vi "Elimina acquisizione.vi"(8 "indice prova":i32, 9 "indice riga":i32, 10 "tabella":i32, 11 "Dati prove in 2":T1) -> (1 "riga eliminata":string[](array[string]), 3 "Dati prove out 3":T1)   [LabVIEW 2019]
uses:
  TypeDef/Dati collaudo.ctl
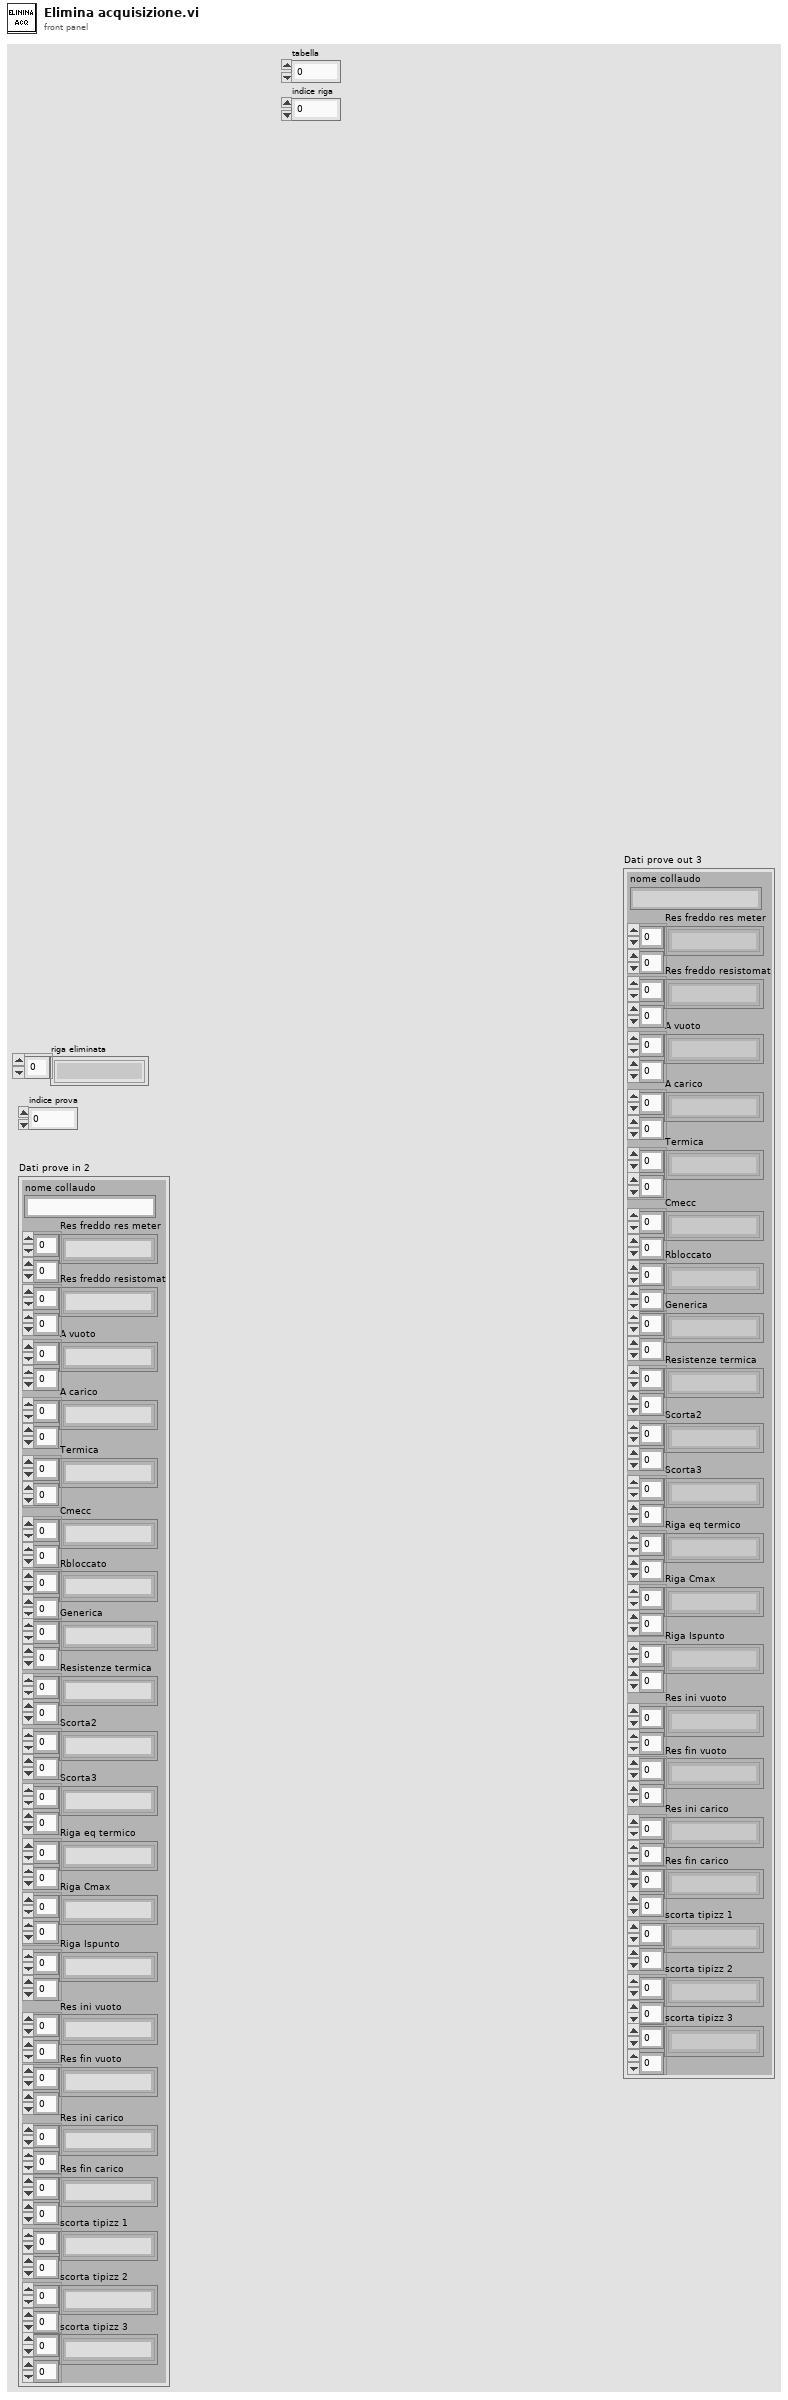
[diagram p1: front panel]
types:
  T1 = typedef "Dati collaudo.ctl" = cluster{"nome collaudo":string, "Res freddo res meter":string[][], "Res freddo resistomat":string[][], "A vuoto":string[][], "A carico":string[][], "Termica":string[][], "Cmecc":string[][], "Rbloccato":string[][], "Generica":string[][], "Resistenze termica":string[][], "Scorta2":string[][], "Scorta3":string[][], "Riga eq termico":string[][], "Riga Cmax":string[][], "Riga Ispunto":string[][], "Res ini vuoto":string[][], "Res fin vuoto":string[][], "Res ini carico":string[][], "Res fin carico":string[][], "scorta tipizz 1":string[][], "scorta tipizz 2":string[][], "scorta tipizz 3":string[][]}
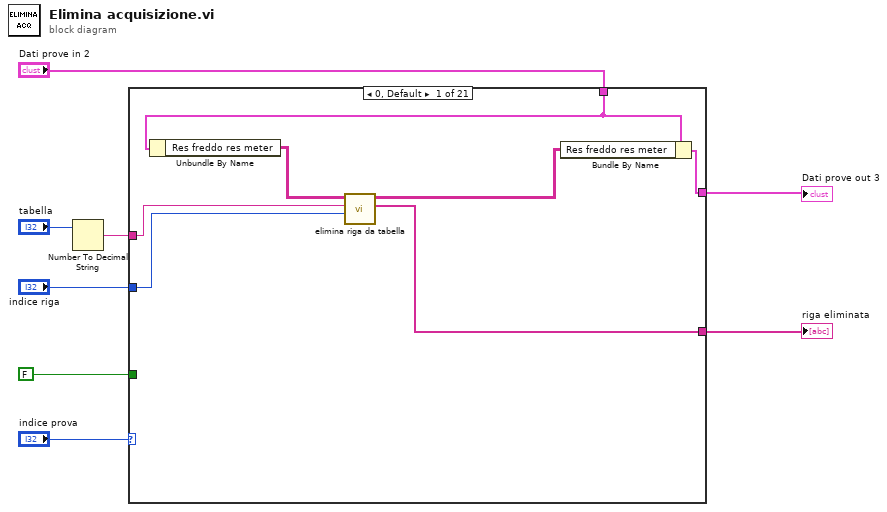
[diagram p0: block diagram]
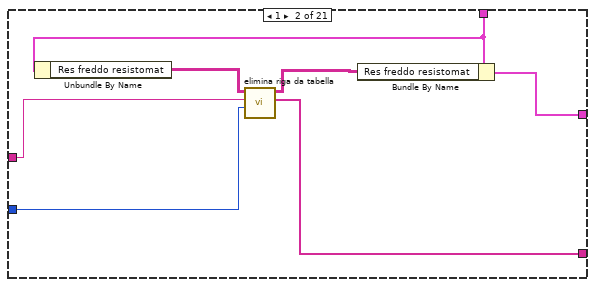
[diagram p2: hidden frame]
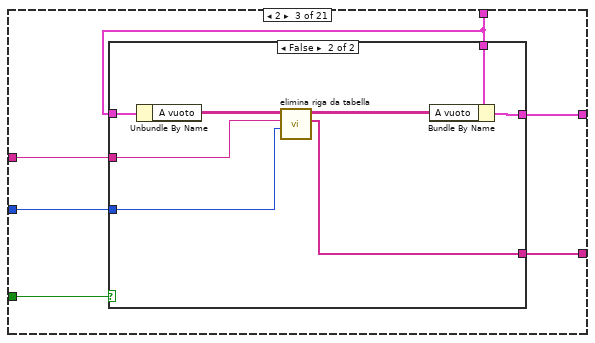
[diagram p3: hidden frame]
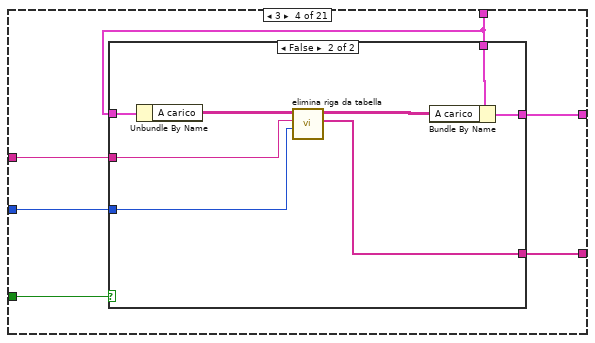
[diagram p5: hidden frame]
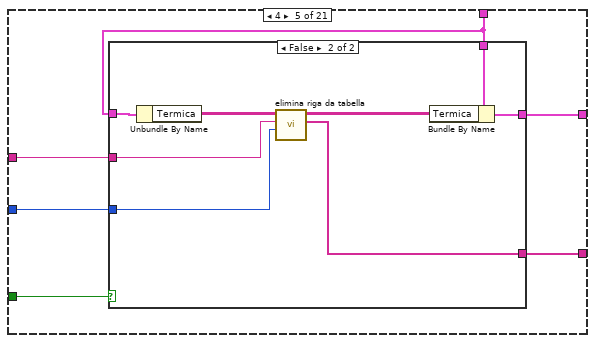
[diagram p7: hidden frame]
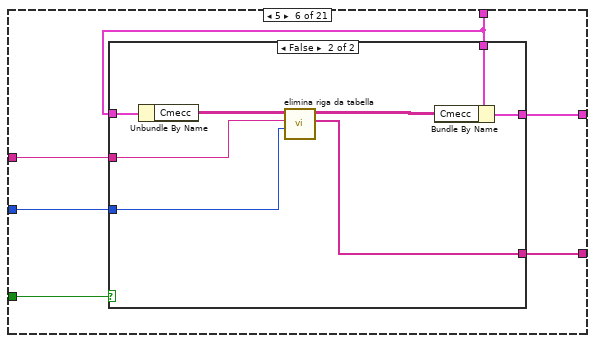
[diagram p9: hidden frame]
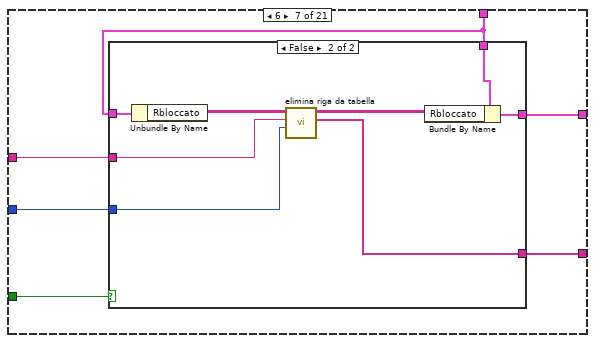
[diagram p11: hidden frame]
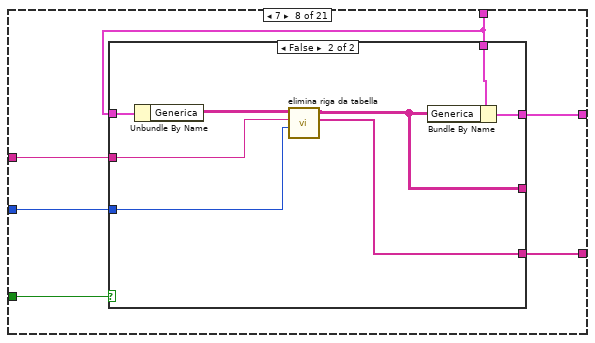
[diagram p13: hidden frame]
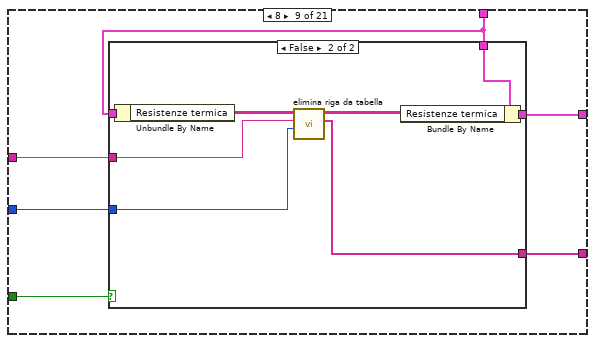
[diagram p15: hidden frame]
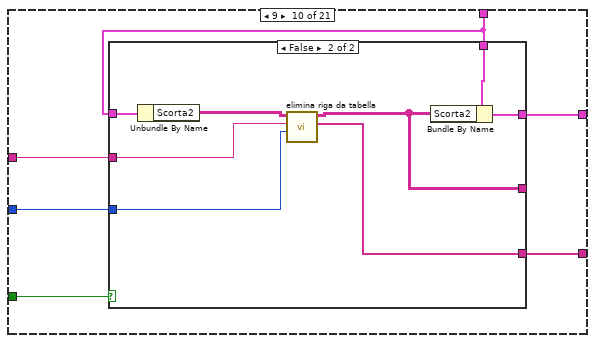
[diagram p17: hidden frame]
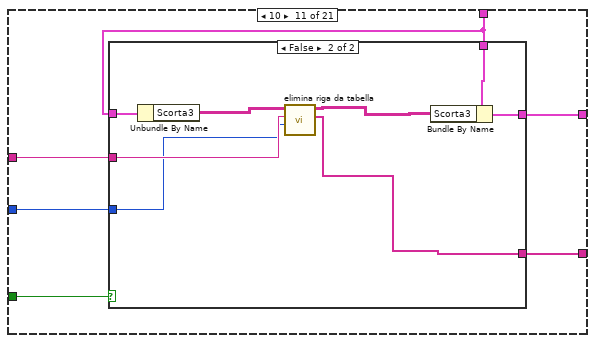
[diagram p19: hidden frame]
diagram:
  n1 = Number To Decimal String(number="tabella") -> (decimal integer string=w3:string)  [unwired: 1 in]
  n2 = case shown="0, Default" "indice prova" {
    tunnel: FALSE -> [_ _ w28 w43 w58 w73 w88 w103 w118 w133 w148 _ _ _ _ _ _ _ _ _ _]
    tunnel: [w15 w22 w27 w42 w57 w72 w87 w102 w117 w132 w147 w164 w171 w178 w185 w192 w199 w206 w213 w220 w227] -> w5
    tunnel: "Dati prove in 2" -> [w14 w21 w26 w41 w56 w71 w86 w101 w116 w131 w146 w163 w170 w177 w184 w191 w198 w205 w212 w219 w226]
    tunnel: [w9 w18 w25 w40 w55 w70 w85 w100 w115 w130 w145 w159 w167 w174 w180 w188 w193 w202 w207 w214 w221] -> w8
    tunnel: w3 -> [w12 w17 w24 w39 w54 w69 w84 w99 w114 w129 w144 w160 w166 w173 w181 w187 w195 w201 w209 w216 w223]
    tunnel: "indice riga" -> [w11 w16 w23 w38 w53 w68 w83 w98 w113 w128 w143 w158 w165 w172 w179 w186 w194 w200 w208 w215 w222]
    frame 0, Default {
      n3 = Unbundle By Name(w14) -> ("Res freddo res meter"=w13:string[][])
      n4 = call "elimina riga da tabella.vi"("indice riga"=w11, "tab"=w12, "Res freddo res meter in"=w13) -> ("riga eliminata"=w9:string[], "Array"=w10:string[][])  [unwired: 7 in]
      n5 = Bundle By Name(cluster=w14, "Res freddo res meter"=w10) -> (w15:T1)
    }
    frame 1 {
      n6 = Unbundle By Name(w21) -> ("Res freddo resistomat"=w20:string[][])
      n7 = call "elimina riga da tabella.vi"("indice riga"=w16, "tab"=w17, "Res freddo res meter in"=w20) -> ("riga eliminata"=w18:string[], "Array"=w19:string[][])  [unwired: 7 in]
      n8 = Bundle By Name(cluster=w21, "Res freddo resistomat"=w19) -> (w22:T1)
    }
    frame 2 {
      n9 = case shown="False" w28 {
        tunnel: [w29 w37] -> w27
        tunnel: w26 -> [w29 w36]
        tunnel: w26 -> [_ w35]
        tunnel: [_ w30] -> w25
        tunnel: w24 -> [_ w32]
        tunnel: w23 -> [_ w31]
        frame True {
        }
        frame False {
          n10 = Unbundle By Name(w35) -> ("A vuoto"=w34:string[][])
          n11 = call "elimina riga da tabella.vi"("indice riga"=w31, "tab"=w32, "Res freddo res meter in"=w34) -> ("riga eliminata"=w30:string[], "Array"=w33:string[][])  [unwired: 7 in]
          n12 = Bundle By Name(cluster=w36, "A vuoto"=w33) -> (w37:T1)
        }
      }
    }
    frame 3 {
      n13 = case shown="False" w43 {
        tunnel: [w44 w52] -> w42
        tunnel: w41 -> [w44 w51]
        tunnel: w41 -> [_ w50]
        tunnel: [_ w45] -> w40
        tunnel: w39 -> [_ w47]
        tunnel: w38 -> [_ w46]
        frame True {
        }
        frame False {
          n14 = Unbundle By Name(w50) -> ("A carico"=w49:string[][])
          n15 = call "elimina riga da tabella.vi"("indice riga"=w46, "tab"=w47, "Res freddo res meter in"=w49) -> ("riga eliminata"=w45:string[], "Array"=w48:string[][])  [unwired: 7 in]
          n16 = Bundle By Name(cluster=w51, "A carico"=w48) -> (w52:T1)
        }
      }
    }
    frame 4 {
      n17 = case shown="False" w58 {
        tunnel: [w59 w67] -> w57
        tunnel: w56 -> [w59 w66]
        tunnel: w56 -> [_ w65]
        tunnel: [_ w60] -> w55
        tunnel: w54 -> [_ w62]
        tunnel: w53 -> [_ w61]
        frame True {
        }
        frame False {
          n18 = Unbundle By Name(w65) -> ("Termica"=w64:string[][])
          n19 = call "elimina riga da tabella.vi"("indice riga"=w61, "tab"=w62, "Res freddo res meter in"=w64) -> ("riga eliminata"=w60:string[], "Array"=w63:string[][])  [unwired: 7 in]
          n20 = Bundle By Name(cluster=w66, "Termica"=w63) -> (w67:T1)
        }
      }
    }
    frame 5 {
      n21 = case shown="False" w73 {
        tunnel: [w74 w82] -> w72
        tunnel: w71 -> [w74 w81]
        tunnel: w71 -> [_ w80]
        tunnel: [_ w75] -> w70
        tunnel: w69 -> [_ w77]
        tunnel: w68 -> [_ w76]
        frame True {
        }
        frame False {
          n22 = Unbundle By Name(w80) -> ("Cmecc"=w79:string[][])
          n23 = call "elimina riga da tabella.vi"("indice riga"=w76, "tab"=w77, "Res freddo res meter in"=w79) -> ("riga eliminata"=w75:string[], "Array"=w78:string[][])  [unwired: 7 in]
          n24 = Bundle By Name(cluster=w81, "Cmecc"=w78) -> (w82:T1)
        }
      }
    }
    frame 6 {
      n25 = case shown="False" w88 {
        tunnel: [w89 w97] -> w87
        tunnel: w86 -> [w89 w96]
        tunnel: w86 -> [_ w95]
        tunnel: [_ w90] -> w85
        tunnel: w84 -> [_ w92]
        tunnel: w83 -> [_ w91]
        frame True {
        }
        frame False {
          n26 = Unbundle By Name(w95) -> ("Rbloccato"=w94:string[][])
          n27 = call "elimina riga da tabella.vi"("indice riga"=w91, "tab"=w92, "Res freddo res meter in"=w94) -> ("riga eliminata"=w90:string[], "Array"=w93:string[][])  [unwired: 7 in]
          n28 = Bundle By Name(cluster=w96, "Rbloccato"=w93) -> (w97:T1)
        }
      }
    }
    frame 7 {
      n29 = case shown="False" w103 {
        tunnel: [_ w108] -> _
        tunnel: [w104 w112] -> w102
        tunnel: w101 -> [w104 w111]
        tunnel: w101 -> [_ w110]
        tunnel: [_ w106] -> w100
        tunnel: w99 -> [_ w107]
        tunnel: w98 -> [_ w105]
        frame True {
        }
        frame False {
          n30 = Unbundle By Name(w110) -> ("Generica"=w109:string[][])
          n31 = call "elimina riga da tabella.vi"("indice riga"=w105, "tab"=w107, "Res freddo res meter in"=w109) -> ("riga eliminata"=w106:string[], "Array"=w108:string[][])  [unwired: 7 in]
          n32 = Bundle By Name(cluster=w111, "Generica"=w108) -> (w112:T1)
        }
      }
    }
    frame 8 {
      n33 = case shown="False" w118 {
        tunnel: [w119 w127] -> w117
        tunnel: w116 -> [w119 w126]
        tunnel: w116 -> [_ w125]
        tunnel: [_ w121] -> w115
        tunnel: w114 -> [_ w122]
        tunnel: w113 -> [_ w120]
        frame True {
        }
        frame False {
          n34 = Unbundle By Name(w125) -> ("Resistenze termica"=w124:string[][])
          n35 = call "elimina riga da tabella.vi"("indice riga"=w120, "tab"=w122, "Res freddo res meter in"=w124) -> ("riga eliminata"=w121:string[], "Array"=w123:string[][])  [unwired: 7 in]
          n36 = Bundle By Name(cluster=w126, "Resistenze termica"=w123) -> (w127:T1)
        }
      }
    }
    frame 9 {
      n37 = case shown="False" w133 {
        tunnel: [_ w138] -> _
        tunnel: [w134 w142] -> w132
        tunnel: w131 -> [w134 w141]
        tunnel: w131 -> [_ w140]
        tunnel: [_ w136] -> w130
        tunnel: w129 -> [_ w137]
        tunnel: w128 -> [_ w135]
        frame True {
        }
        frame False {
          n38 = Unbundle By Name(w140) -> ("Scorta2"=w139:string[][])
          n39 = call "elimina riga da tabella.vi"("indice riga"=w135, "tab"=w137, "Res freddo res meter in"=w139) -> ("riga eliminata"=w136:string[], "Array"=w138:string[][])  [unwired: 7 in]
          n40 = Bundle By Name(cluster=w141, "Scorta2"=w138) -> (w142:T1)
        }
      }
    }
    frame 10 {
      n41 = case shown="False" w148 {
        tunnel: [w149 w157] -> w147
        tunnel: w146 -> [w149 w156]
        tunnel: w146 -> [_ w155]
        tunnel: [_ w151] -> w145
        tunnel: w144 -> [_ w152]
        tunnel: w143 -> [_ w150]
        frame True {
        }
        frame False {
          n42 = Unbundle By Name(w155) -> ("Scorta3"=w154:string[][])
          n43 = call "elimina riga da tabella.vi"("indice riga"=w150, "tab"=w152, "Res freddo res meter in"=w154) -> ("riga eliminata"=w151:string[], "Array"=w153:string[][])  [unwired: 7 in]
          n44 = Bundle By Name(cluster=w156, "Scorta3"=w153) -> (w157:T1)
        }
      }
    }
    frame 11 {
      n45 = Unbundle By Name(w163) -> ("Riga eq termico"=w162:string[][])
      n46 = call "elimina riga da tabella.vi"("indice riga"=w158, "tab"=w160, "Res freddo res meter in"=w162) -> ("riga eliminata"=w159:string[], "Array"=w161:string[][])  [unwired: 7 in]
      n47 = Bundle By Name(cluster=w163, "Riga eq termico"=w161) -> (w164:T1)
    }
    frame 12 {
      n48 = Unbundle By Name(w170) -> ("Riga Cmax"=w169:string[][])
      n49 = call "elimina riga da tabella.vi"("indice riga"=w165, "tab"=w166, "Res freddo res meter in"=w169) -> ("riga eliminata"=w167:string[], "Array"=w168:string[][])  [unwired: 7 in]
      n50 = Bundle By Name(cluster=w170, "Riga Cmax"=w168) -> (w171:T1)
    }
    frame 13 {
      n51 = Unbundle By Name(w177) -> ("Riga Ispunto"=w176:string[][])
      n52 = call "elimina riga da tabella.vi"("indice riga"=w172, "tab"=w173, "Res freddo res meter in"=w176) -> ("riga eliminata"=w174:string[], "Array"=w175:string[][])  [unwired: 7 in]
      n53 = Bundle By Name(cluster=w177, "Riga Ispunto"=w175) -> (w178:T1)
    }
    frame 14 {
      n54 = Unbundle By Name(w184) -> ("Res ini vuoto"=w183:string[][])
      n55 = call "elimina riga da tabella.vi"("indice riga"=w179, "tab"=w181, "Res freddo res meter in"=w183) -> ("riga eliminata"=w180:string[], "Array"=w182:string[][])  [unwired: 7 in]
      n56 = Bundle By Name(cluster=w184, "Res ini vuoto"=w182) -> (w185:T1)
    }
    frame 15 {
      n57 = Unbundle By Name(w191) -> ("Res fin vuoto"=w190:string[][])
      n58 = call "elimina riga da tabella.vi"("indice riga"=w186, "tab"=w187, "Res freddo res meter in"=w190) -> ("riga eliminata"=w188:string[], "Array"=w189:string[][])  [unwired: 7 in]
      n59 = Bundle By Name(cluster=w191, "Res fin vuoto"=w189) -> (w192:T1)
    }
    frame 16 {
      n60 = Unbundle By Name(w198) -> ("Res ini carico"=w197:string[][])
      n61 = call "elimina riga da tabella.vi"("indice riga"=w194, "tab"=w195, "Res freddo res meter in"=w197) -> ("riga eliminata"=w193:string[], "Array"=w196:string[][])  [unwired: 7 in]
      n62 = Bundle By Name(cluster=w198, "Res ini carico"=w196) -> (w199:T1)
    }
    frame 17 {
      n63 = Unbundle By Name(w205) -> ("Res fin carico"=w204:string[][])
      n64 = call "elimina riga da tabella.vi"("indice riga"=w200, "tab"=w201, "Res freddo res meter in"=w204) -> ("riga eliminata"=w202:string[], "Array"=w203:string[][])  [unwired: 7 in]
      n65 = Bundle By Name(cluster=w205, "Res fin carico"=w203) -> (w206:T1)
    }
    frame 18 {
      n66 = Unbundle By Name(w212) -> ("scorta tipizz 1"=w211:string[][])
      n67 = call "elimina riga da tabella.vi"("indice riga"=w208, "tab"=w209, "Res freddo res meter in"=w211) -> ("riga eliminata"=w207:string[], "Array"=w210:string[][])  [unwired: 7 in]
      n68 = Bundle By Name(cluster=w212, "scorta tipizz 1"=w210) -> (w213:T1)
    }
    frame 19 {
      n69 = Unbundle By Name(w219) -> ("scorta tipizz 2"=w218:string[][])
      n70 = call "elimina riga da tabella.vi"("indice riga"=w215, "tab"=w216, "Res freddo res meter in"=w218) -> ("riga eliminata"=w214:string[], "Array"=w217:string[][])  [unwired: 7 in]
      n71 = Bundle By Name(cluster=w219, "scorta tipizz 2"=w217) -> (w220:T1)
    }
    frame 20 {
      n72 = Unbundle By Name(w226) -> ("scorta tipizz 3"=w225:string[][])
      n73 = call "elimina riga da tabella.vi"("indice riga"=w222, "tab"=w223, "Res freddo res meter in"=w225) -> ("riga eliminata"=w221:string[], "Array"=w224:string[][])  [unwired: 7 in]
      n74 = Bundle By Name(cluster=w226, "scorta tipizz 3"=w224) -> (w227:T1)
    }
  }
  "Dati prove out 3" <- w5
  "riga eliminata" <- w8
